vi "icListen 3 Enabled.vi"() -> ()   [LabVIEW 2020, in "PAM Library.lvlib"]
uses:
  PAM Library.lvlib
panel:
  in  "icLsiten 3 Enabled":bool
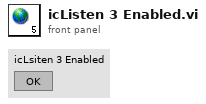
[diagram p1: front panel]
diagram:
